vi "Type Paths OoC.vi"() -> (0 "error out":errorcluster, 2 "Type Path Map":map{path, path}(c390))   [LabVIEW 2020, in "Conditum-Tools.lvlib" / "Entity Editor.lvclass"]
uses:
  Entity Editor.lvclass
  <vilib>/IlluminatedG/IG Conditum Base/Conditum/Columns/Boolean/Boolean.lvclass
  C:/Program Files (x86)/National Instruments/LabVIEW 2020/vi.lib/IlluminatedG/IG Conditum Base/Conditum/Columns/Type/Type.lvclass
  <vilib>/IlluminatedG/IG Conditum Base/Conditum/Columns/Double/Double.lvclass
  <vilib>/IlluminatedG/IG Conditum Base/Conditum/Columns/Entity Collection/Entity Collection.lvclass
  <vilib>/IlluminatedG/IG Conditum Base/Conditum/Columns/Entity/Entity.lvclass
  <vilib>/IlluminatedG/IG Conditum Base/Conditum/Columns/ID/ID.lvclass
  <vilib>/IlluminatedG/IG Conditum Base/Conditum/Columns/Integer/Integer.lvclass
  <vilib>/IlluminatedG/IG Conditum Base/Conditum/Columns/String/String.lvclass
  <vilib>/IlluminatedG/IG Conditum Base/Conditum/Columns/Text/Text.lvclass
  <vilib>/IlluminatedG/IG Conditum Base/Conditum/Columns/Timestamp/Timestamp.lvclass
  Conditum-Clone/Columns/Boolean/Boolean.lvclass
  C:/dev/lv20CE/lv-conditum-tools/Conditum-Clone/Columns/Type/Type.lvclass
  Conditum-Clone/Columns/Double/Double.lvclass
  Conditum-Clone/Columns/Entity Collection/Entity Collection.lvclass
  Conditum-Clone/Columns/Entity/Entity.lvclass
  Conditum-Clone/Columns/ID/ID.lvclass
  Conditum-Clone/Columns/Integer/Integer.lvclass
  Conditum-Clone/Columns/String/String.lvclass
  Conditum-Clone/Columns/Text/Text.lvclass
  Conditum-Clone/Columns/Timestamp/Timestamp.lvclass
  Conditum-Tools.lvlib
  Conditum-Clone/Columns/Type/Type.lvclass
  <vilib>/IlluminatedG/IG Conditum Base/Conditum/Columns/Type/Type.lvclass
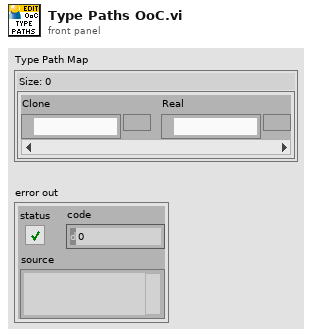
[diagram p1: front panel]
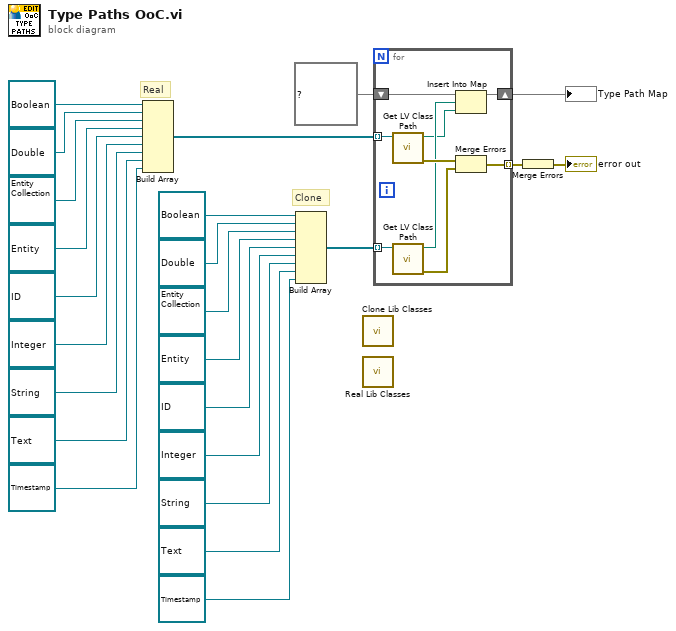
[diagram p0: block diagram]
diagram:
  # "Clone"
  # "Real"
  n1 = Build Array(refnum<class "Boolean.lvclass"> refnum ("Conditum:Columns:Boolean.lvclass"), refnum<class "Double.lvclass"> refnum ("Conditum:Columns:Double.lvclass"), refnum<class "Entity Collection.lvclass"> refnum ("Conditum:Columns:Entity Collection.lvclass"), refnum<class "Entity.lvclass"> refnum ("Conditum:Columns:Entity.lvclass"), refnum<class "ID.lvclass"> refnum ("Conditum:Columns:ID.lvclass"), refnum<class "Integer.lvclass"> refnum ("Conditum:Columns:Integer.lvclass"), refnum<class "String.lvclass"> refnum ("Conditum:Columns:String.lvclass"), refnum<class "Text.lvclass"> refnum ("Conditum:Columns:Text.lvclass"), refnum<class "Timestamp.lvclass"> refnum ("Conditum:Columns:Timestamp.lvclass")) -> (w5:refnum<class "Type.lvclass">[])
  n2 = Build Array(refnum<class "Boolean.lvclass"> refnum ("Conditum:Columns:Boolean.lvclass"), refnum<class "Double.lvclass"> refnum ("Conditum:Columns:Double.lvclass"), refnum<class "Entity Collection.lvclass"> refnum ("Conditum:Columns:Entity Collection.lvclass"), refnum<class "Entity.lvclass"> refnum ("Conditum:Columns:Entity.lvclass"), refnum<class "ID.lvclass"> refnum ("Conditum:Columns:ID.lvclass"), refnum<class "Integer.lvclass"> refnum ("Conditum:Columns:Integer.lvclass"), refnum<class "String.lvclass"> refnum ("Conditum:Columns:String.lvclass"), refnum<class "Text.lvclass"> refnum ("Conditum:Columns:Text.lvclass"), refnum<class "Timestamp.lvclass"> refnum ("Conditum:Columns:Timestamp.lvclass")) -> (w6:refnum<class "Type.lvclass">[])
  n3 = call "Clone Lib Classes.vi"() -> ()  [unwired: 12 in]
  n4 = call "Real Lib Classes.vi"() -> ()  [unwired: 12 in]
  n5 = for {
    tunnel: w6 -> [w31] mode=indexing
    tunnel: w5 -> [w32] mode=indexing
    shift-right: [w27] -> w1
    shift-left: map{path, path} {} ("Type Path Map") -> [w30]
    tunnel: [w25] -> w3 mode=indexing
    n6 = call <vilib>:"Get LV Class Path.vi"("object"=w32) -> ("error out"=w33:errorcluster, "class path"=w28:path)  [unwired: 9 in]
    n7 = call <vilib>:"Get LV Class Path.vi"("object"=w31) -> ("error out"=w26:errorcluster, "class path"=w29:path)  [unwired: 9 in]
    n8 = Insert Into Map(map in=w30, key=w29, value=w28) -> (map out=w27:map{path, path})  [unwired: 2 out]
    n9 = Merge Errors(w33, w26) -> (w25:errorcluster)
  }
  "Type Path Map" <- w1
  n10 = Merge Errors(w3) -> (→"error out":errorcluster)
